vi "Truncation.vi"(0 "original signals":cdb[](array[numeric]) caption="Original signal" format="%.2f", 5 "Samples Per Symbol (16)":i32=16, 7 "Number of Symbols":i32, 9 "TX Pulse Shaping Filter Coefficients":dbl[](array[numeric]) format="%.2f", 11 "RX Matched Filter Coefficients":dbl[](array[numeric]) format="%.2f", 12 "Truncation?":bool=TRUE) -> (4 "truncated signals":cdb[](array[numeric]) caption="Truncated signal" format="%.2f")   [LabVIEW 2011]
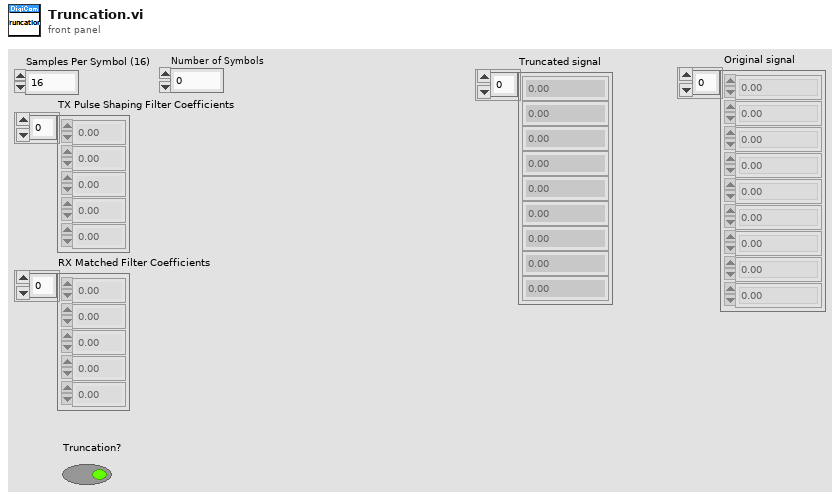
[diagram p1: front panel]
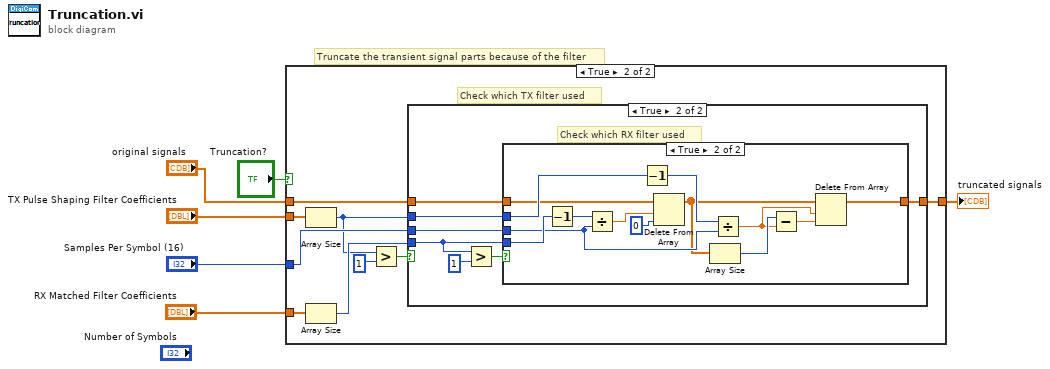
[diagram p0: block diagram]
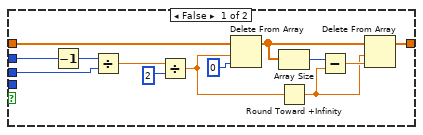
[diagram p4: hidden frame]
diagram:
  # "Truncate the transient signal parts because of the filter"
  n1 = case shown="True" "Truncation?" {
    tunnel: "original signals" -> [w7 w12]
    tunnel: [w7 w11] -> w4
    tunnel: "TX Pulse Shaping Filter Coefficients" -> [_ w10]
    tunnel: "RX Matched Filter Coefficients" -> [_ w16]
    tunnel: "Samples Per Symbol (16)" -> [_ w9]
    frame False {
    }
    frame True {
      # "Check which TX filter used"
      n2 = Array Size(array=w10) -> (size(s)=w8:i32)
      n3 = Array Size(array=w16) -> (size(s)=w13:i32)
      n4 = Greater?(x=w8, y=1) -> (0:w14:bool)
      n5 = case shown="True" w14 {
        tunnel: w13 -> [_ w22]
        tunnel: w12 -> [w17 w19]
        tunnel: [w17 w18] -> w11
        tunnel: w9 -> [_ w21]
        tunnel: w8 -> [_ w20]
        frame False {
        }
        frame True {
          # "Check which RX filter used"
          n6 = Greater?(x=w22, y=1) -> (0:w23:bool)
          n7 = case shown="True" w23 {
            tunnel: w22 -> [_ w50]
            tunnel: w21 -> [w35 w46]
            tunnel: w20 -> [w25 w49]
            tunnel: w19 -> [w34 w45]
            tunnel: [w28 w41] -> w18
            frame False {
              n8 = Decrement(x=w25) -> (x-1=w36:i32)
              n9 = Divide(x=w36, y=w35) -> (x/y=w33:dbl)
              n10 = Divide(x=w33, y=2) -> (x/y=w27:dbl)
              n11 = Delete From Array(array=w34, length=w27, index=0) -> (array with subset deleted=w30:cdb[])  [unwired: 1 out]
              n12 = Array Size(array=w30) -> (size(s)=w29:i32)
              n13 = Round Toward +Infinity(x=w27) -> (ceil(x): smallest int >= x=w26:dbl)
              n14 = Subtract(x=w29, y=w26) -> (x-y=w31:dbl)
              n15 = Delete From Array(array=w30, length=w26, index=w31) -> (array with subset deleted=w28:cdb[])  [unwired: 1 out]
            }
            frame True {
              n16 = Decrement(x=w50) -> (x-1=w48:i32)
              n17 = Divide(x=w48, y=w46) -> (x/y=w44:dbl)
              n18 = Decrement(x=w49) -> (x-1=w47:i32)
              n19 = Delete From Array(array=w45, length=w44, index=0) -> (array with subset deleted=w42:cdb[])  [unwired: 1 out]
              n20 = Array Size(array=w42) -> (size(s)=w39:i32)
              n21 = Divide(x=w47, y=w46) -> (x/y=w38:dbl)
              n22 = Subtract(x=w39, y=w38) -> (x-y=w40:dbl)
              n23 = Delete From Array(array=w42, length=w38, index=w40) -> (array with subset deleted=w41:cdb[])  [unwired: 1 out]
            }
          }
        }
      }
    }
  }
  "truncated signals" <- w4
